vi "Points Collection.vi"() -> (3 "RefPointsColl":refnum<k24>)   [LabVIEW 2021, in "NMEA_GPS Ublox M8N.lvlib"]
uses:
  NMEA_GPS Ublox M8N.lvlib
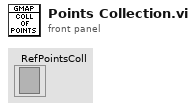
[diagram p1: front panel]
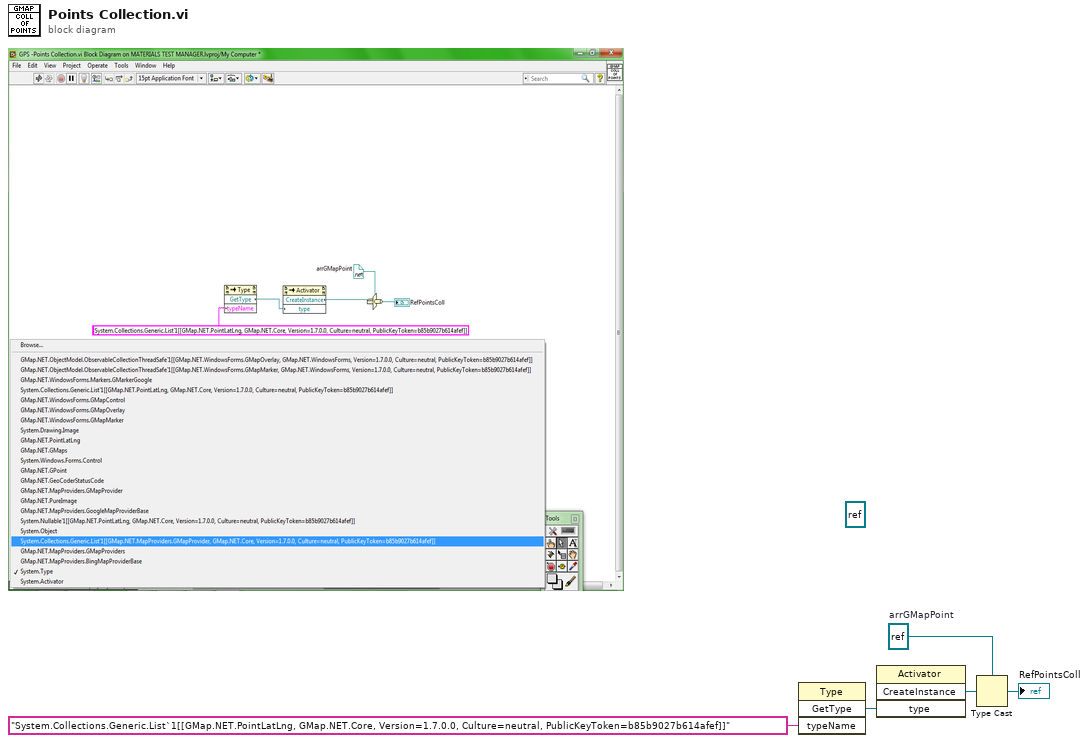
[diagram p0: block diagram]
diagram:
  (unwired) refnum<k24> refnum ("points")
  w3 = refnum<k24> refnum  # arrGMapPoint
  n1 = invoke class="Type" method="GetType"("typeName"="System.Collections.Generic.List`1[[GMap.NET.PointLatLng, GMap.NET.Core, Version=1.7.0.0, Culture=neutral, PublicKeyToken=b85b9027b614afef]]") -> ("GetType"=w1:refnum<k24>)  [unwired: 3 in, 3 out]
  n2 = invoke class="Activator" method="CreateInstance"("type"=w1) -> ("CreateInstance"=w2:refnum<k24>)  [unwired: 3 in, 3 out]
  n3 = Type Cast(type=w3, x=w2) -> (*(type *) &x=→"RefPointsColl":refnum<k24>)
